vi "Get PDOMapping.vi"(8 "error in":errorcluster, 11 "Object Type in":refnum<class "Object Type Base.lvclass">) -> (0 "error out":errorcluster, 1 "Defined?":bool, 2 "PDOMapping":bool, 3 "Object Type out":refnum<class "Object Type Base.lvclass">)   [LabVIEW 2019, in "Electronic Datasheet.lvlib" / "Object Type Base.lvclass"]
uses:
  Object Type Base.lvclass
  Object Type Base.lvclass/Object Type Base.ctl
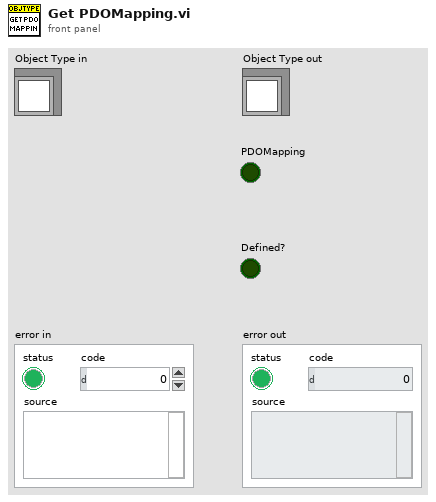
[diagram p1: front panel]
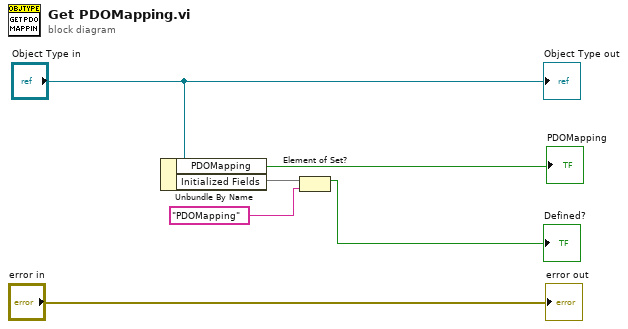
[diagram p0: block diagram]
diagram:
  n1 = Unbundle By Name("Object Type in") -> ("PDOMapping"=→"PDOMapping":bool, "Initialized Fields"=w5:set{string})
  n2 = Element of Set?(10:"PDOMapping" ("element"), 11:w5) -> (3:→"Defined?":bool)
  "Object Type out" <- "Object Type in"
  "error out" <- "error in"
